vi "get channels.vi"(11 "Shared Memory configuration in":refnum<class "Shared Memory configuration.lvclass">) -> (2 "channels":refnum<class "TBM channel.lvclass">[](array[class]), 3 "Shared Memory configuration out":refnum<class "Shared Memory configuration.lvclass">)   [LabVIEW 2013, in "Shared Memory configuration.lvclass"]
doc: "Returns an array of all Channels currently added to this configuration object."
uses:
  Shared Memory configuration.lvclass
  <vilib>/NI/Tag Bus Module Framework/channel/TBM channel.lvclass
  Shared Memory configuration.lvclass/Shared Memory configuration.ctl
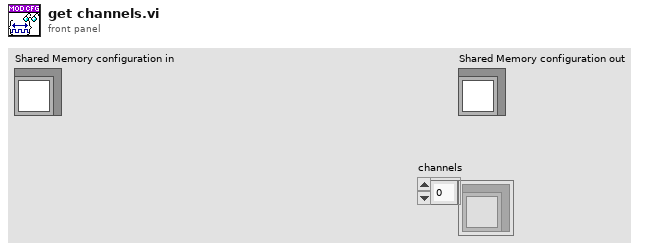
[diagram p1: front panel]
types:
  T1 = typedef "Shared Memory configuration.lvclass/Line.ctl" = cluster{"channel":refnum<class "TBM channel.lvclass">}
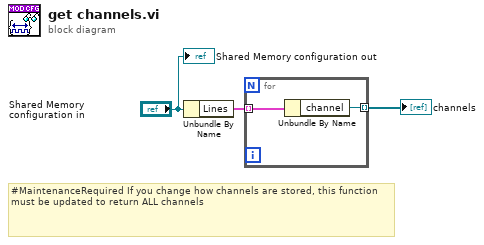
[diagram p0: block diagram]
diagram:
  # "#MaintenanceRequired If you change how channels are stored, this function must be updated to return ALL channels"
  n1 = Unbundle By Name("Shared Memory configuration in") -> ("Lines"=w2:T1[])
  n2 = for {
    tunnel: w2 -> [w5] mode=indexing
    tunnel: [w4] -> w1 mode=indexing
    n3 = Unbundle By Name(w5) -> ("channel"=w4:refnum<class "TBM channel.lvclass">)
  }
  "channels" <- w1
  "Shared Memory configuration out" <- "Shared Memory configuration in"
